vi "Close.vi"(8 "error in":errorcluster, 11 "Message Buffer in":refnum<class "Message Buffer.lvclass">) -> (0 "error out":errorcluster, 3 "Message Buffer out":refnum<class "Message Buffer.lvclass">)   [LabVIEW 2024, in "PCAN.lvlib" / "Message Buffer.lvclass"]
uses:
  Message Buffer.lvclass
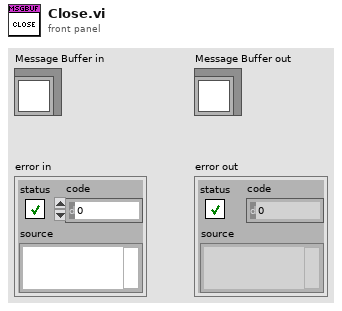
[diagram p1: front panel]
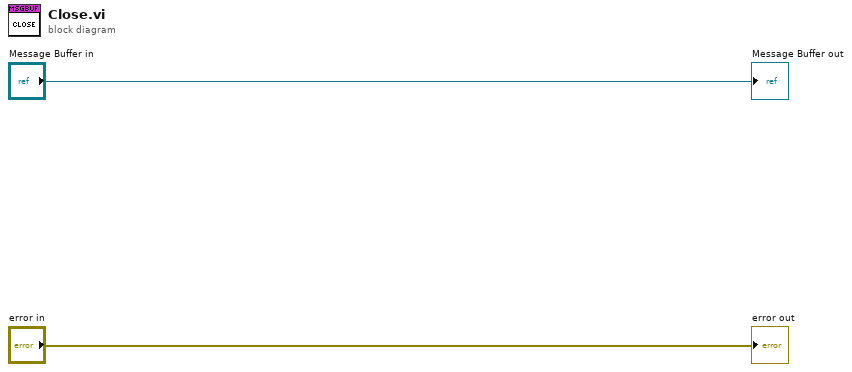
[diagram p0: block diagram]
diagram:
  "error out" <- "error in"
  "Message Buffer out" <- "Message Buffer in"
